vi "Rundenzeit.vi"(11 "8 IR true":bool) -> (3 "Rundenzeiten":dbl[](array[numeric])=[inf, inf, inf, inf, inf, inf, inf])   [LabVIEW 2016]
panel:
  # "Minimum"
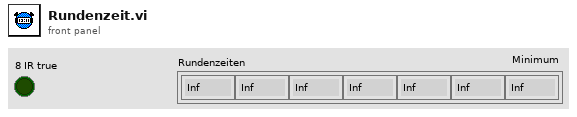
[diagram p1: front panel]
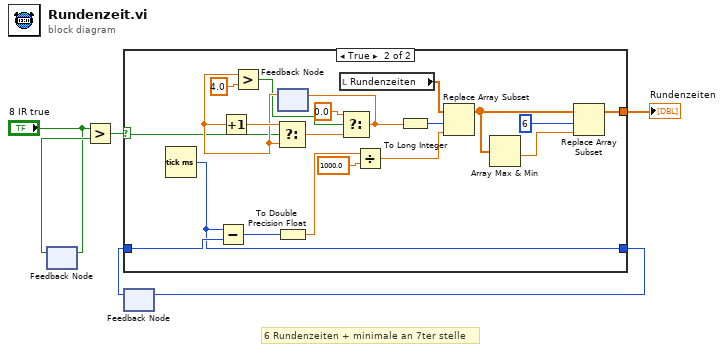
[diagram p0: block diagram]
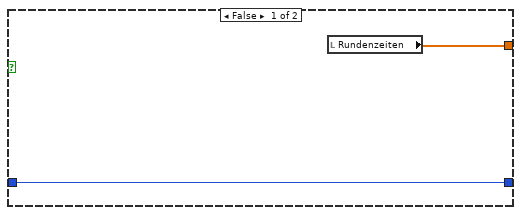
[diagram p2: hidden frame]
diagram:
  # "6 Rundenzeiten + minimale an 7ter stelle"
  n1 = feedback #1() -> (w4:bool)  [unwired: 1 in]
  n2 = feedback-in #1("8 IR true") -> ()
  n3 = Greater?(x="8 IR true", y=w4) -> (0:w3:bool)
  n4 = feedback #2() -> (w5:u32)  [unwired: 1 in]
  n5 = case shown="True" w3 {
    selector: w3 -> [_ w16]
    tunnel: [w8 w24] -> w6
    tunnel: w5 -> [w8 w28]
    tunnel: [w7 w12] -> w1
    frame False {
      n6 = local read "Rundenzeiten"() -> (w7:dbl[])
    }
    frame True {
      n7 = Tick Count (ms)() -> (millisecond timer value=w24:u32)
      n8 = Subtract(x=w24, y=w28) -> (x-y=w25:u32)
      n9 = feedback #3() -> (w19:dbl)  [unwired: 1 in]
      n10 = Increment(x=w19) -> (x+1=w21:dbl)
      n11 = Greater?(x=w19, y=4.0) -> (0:w18:bool)
      n12 = Select(t=w21, s=w16, f=w19) -> (s? t:f=w20:dbl)
      n13 = To Double Precision Float(number=w25) -> (double precision float=w27:dbl)
      n14 = local read "Rundenzeiten"() -> (w22:dbl[])
      n15 = Select(t=0.0, s=w18, f=w20) -> (s? t:f=w13:dbl)
      n16 = feedback-in #3(w13) -> ()
      n17 = Divide(x=w27, y=1000.0) -> (x/y=w23:dbl)
      n18 = To Long Integer(number=w13) -> (32bit integer=w14:i32)
      n19 = Replace Array Subset(array=w22, new element=w23, index=w14) -> (w10:dbl[])
      n20 = Array Max & Min(array=w10) -> (min value=w9:dbl)  [unwired: 3 out]
      n21 = Replace Array Subset(array=w10, new element=w9, index=6) -> (w12:dbl[])
    }
  }
  "Rundenzeiten" <- w1
  n22 = feedback-in #2(w6) -> ()
